vi "Framework.Increment Plugins.vi"(8 "error in (no error)":errorcluster, 11 "Framework in":refnum<class "Framework.lvclass">) -> (0 "error out":errorcluster, 3 "Framework out":refnum<class "Framework.lvclass">)   [LabVIEW 2017, in "DSF Core.lvlib" / "Framework.lvclass"]
uses:
  Framework.lvclass
  Framework.lvclass/Framework.ctl
  Plugin/Plugin.lvclass/Plugin.ctl
  Timing/Timing.lvclass/Timing.ctl
  Timing/Increment Iteration.vi
  Plugin/Plugin.Get Timing.vi
  Timing/Is Active Cycle.vi
  Timing/Get Decimation.vi
  Timing/Get Offset.vi
  Plugin/Plugin.lvclass
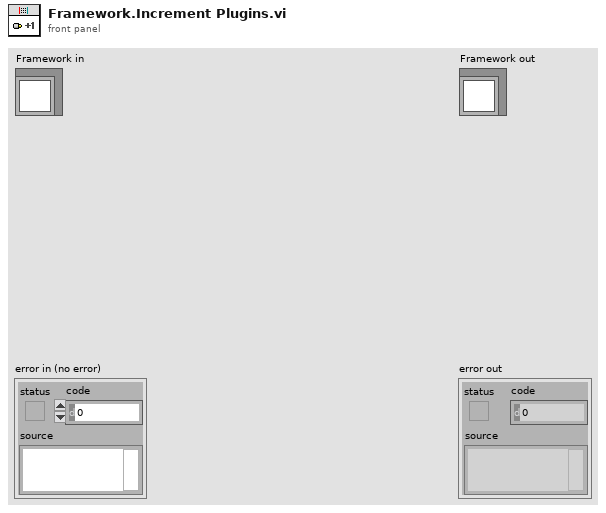
[diagram p1: front panel]
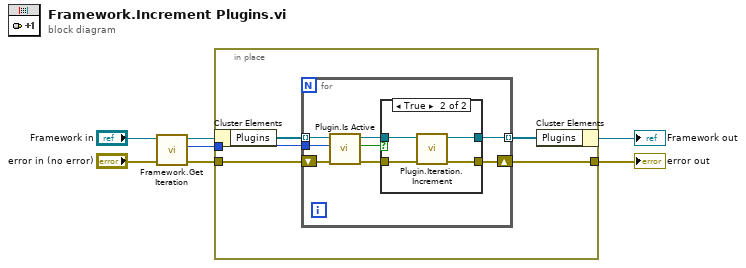
[diagram p0: block diagram]
diagram:
  n1 = call "Framework.Get Iteration.vi"("Framework in"="Framework in") -> ("iteration"=w4:u64, "Framework out"=w1:refnum<class "Framework.lvclass">)  [unwired: 9 in]
  n2 = in-place {
    in-place-border: [w11] -> w6
    in-place-border: "error in (no error)" -> [w10]
    in-place-border: w4 -> [w9]
    n3 = in-place-cluster #1(w1) -> ("Plugins"=w8:refnum<class "Plugin.lvclass">[])
    n4 = for {
      tunnel: w8 -> [w15] mode=indexing
      tunnel: [w18] -> w7 mode=indexing
      shift-right: [w17] -> w11
      shift-left: w10 -> [w16]
      tunnel: w9 -> [w12]
      n5 = call "Plugin.Is Active.vi"("cycle count"=w12, "Plugin in"=w15) -> ("active this cycle?"=w13:bool, "Plugin out"=w14:refnum<class "Plugin.lvclass">)  [unwired: 8 in]
      n6 = case shown="True" w13 {
        tunnel: [w19 w24] -> w18
        tunnel: [w20 w23] -> w17
        tunnel: w16 -> [w20 w22]
        tunnel: w14 -> [w19 w21]
        frame False {
        }
        frame True {
          n7 = call "Plugin.Iteration.Increment.vi"("error in (no error)"=w22, "Plugin in"=w21) -> ("error out"=w23:errorcluster, "Plugin out"=w24:refnum<class "Plugin.lvclass">)  [unwired: 8 in]
        }
      }
    }
    n8 = in-place-cluster #1("Plugins"=w7) -> (→"Framework out":refnum<class "Framework.lvclass">)
  }
  "error out" <- w6
